vi "温湿度告警字符串组合 (子VI).vi"(9 "AD01":sgl, 10 "室温湿度上限告警点":dbl, 11 "室温湿度下限告警点":dbl) -> (3 "字符串":string="正常")   [LabVIEW 2016, in "环境动力监测库.lvlib"]
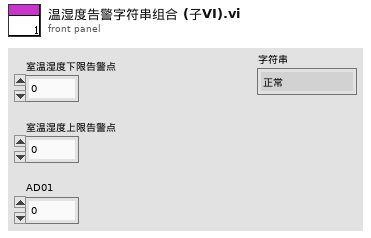
[diagram p1: front panel]
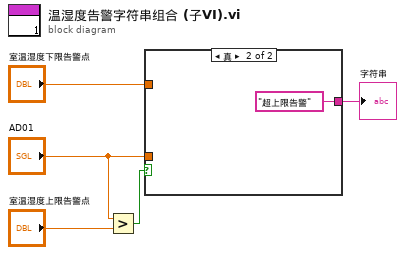
[diagram p0: block diagram]
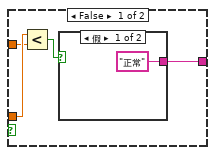
[diagram p2: hidden frame]
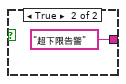
[diagram p3: hidden frame]
diagram:
  n1 = Greater?(x="AD01", y="室温湿度上限告警点") -> (0:w5:bool)
  n2 = case shown="真" w5 {
    tunnel: "AD01" -> [w9 _]
    tunnel: "室温湿度下限告警点" -> [w8 _]
    tunnel: [w6 "超上限告警"] -> w1
    frame False {
      n3 = Less?(x=w9, y=w8) -> (x < y?=w7:bool)
      n4 = case shown="假" w7 {
        tunnel: ["正常" "超下限告警"] -> w6
        frame False {
        }
        frame True {
        }
      }
    }
    frame True {
    }
  }
  "字符串" <- w1
